vi "TCPreadTerminatedString.vi"(8 "error in (no error)":errorcluster, 11 "TCP Network Connection in":refnum<k5>) -> (0 "error out":errorcluster, 2 "string out":string, 3 "TCP Network Connection out":refnum<k5>)   [LabVIEW 2014]
doc: "Read the tcp striam until a full string terminated by CRLF is received. ITo allow very long strings, instead of using an oversized input buffer, grow the string in LV memory by concatenating chunks in a while loop."
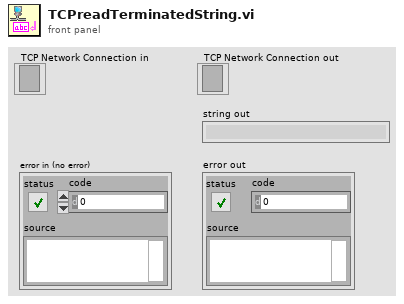
[diagram p1: front panel]
types:
  T1 = enum16{"Standard", "Buffered", "CRLF", "Immediate"}
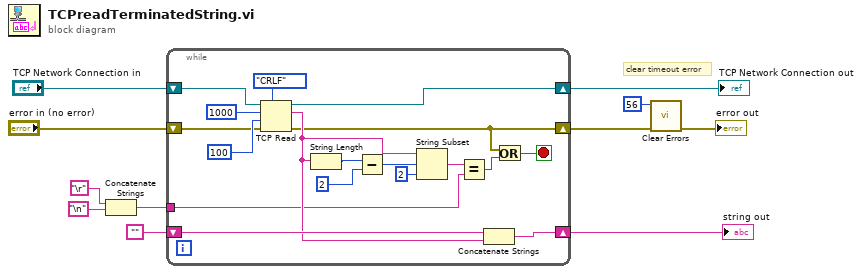
[diagram p0: block diagram]
diagram:
  # "clear timeout error"
  n1 = Concatenate Strings("\r", "\n") -> (w1:string)
  n2 = while {
    shift-right: [w13] -> w9
    shift-left: "error in (no error)" -> [w26]
    shift-right: [w25] -> w7
    shift-left: "TCP Network Connection in" -> [w24]
    shift-right: [w22] -> w2
    shift-left: "" -> [w23]
    tunnel: w1 -> [w15]
    stop <- w12 stop-if-true
    n3 = TCP Read(connection ID=w24, bytes to read=1000, error in (no error)=w26, 7:T1."CRLF" ("mode (standard)"), 9:100 ("timeout ms (25000)")) -> (connection ID out=w25:refnum<k5>, data out=w17:string, error out=w13:errorcluster)
    n4 = String Length(string=w17) -> (length=w21:i32)
    n5 = Subtract(x=w21, y=2 ("x")) -> (x-y=w19:i32)
    n6 = String Subset(string=w17, offset (0)=w19, length (rest)=2 ("length (rest)")) -> (substring=w16:string)
    n7 = Equal?(x=w16, y=w15) -> (x = y?=w14:bool)
    n8 = Concatenate Strings(w23, w17) -> (w22:string)
    n9 = Or(x=w13, y=w14) -> (x .or. y?=w12:bool)
  }
  "string out" <- w2
  "TCP Network Connection out" <- w7
  n10 = call <vilib>:"Clear Errors.vi"("error in (no error)"=w9, "specific error code to clear (0: all)"=56) -> ("error out"=→"error out":errorcluster)  [unwired: 4 in, 1 out]
